vi "DAQ-Data-to-File Load Configuration Settings from XML.vi"(8 "error in (no error)":errorcluster, 11 "User Configuration in":T1={"Hardware Configuration"={"HW Refnum <Replace Me>"="", "Signal Type <Replace Me>"=enum."Sine Wave"}, "Analysis Configuration"={"Statistics"=TRUE}, "New Data Behavior"=enum."Replace"}) -> (0 "error out":errorcluster, 3 "User Configuration out":T1={"Hardware Configuration"={"HW Refnum <Replace Me>"="", "Signal Type <Replace Me>"=enum."Sine Wave"}, "Analysis Configuration"={"Statistics"=TRUE}, "New Data Behavior"=enum."Replace"})   [LabVIEW 2020]
doc: "Attempts to load previous user specified settings from an XML file.\n\nThis VI will not generate an error. If a suitable XML file can't be loaded and parsed then it will simply return the default settings."
uses:
  controls/DAQ-Data-to-File User Specified Data.ctl
  controls/DAQ-Data-to-File HW Configuration.ctl
  controls/DAQ-Data-to-File Simulated Signal Type.ctl
  controls/DAQ-Data-to-File Analysis Configuration.ctl
  controls/DAQ-Data-to-File New Data Behavior.ctl
  <vilib>/Utility/xml.llb/Read From XML File(string).vi
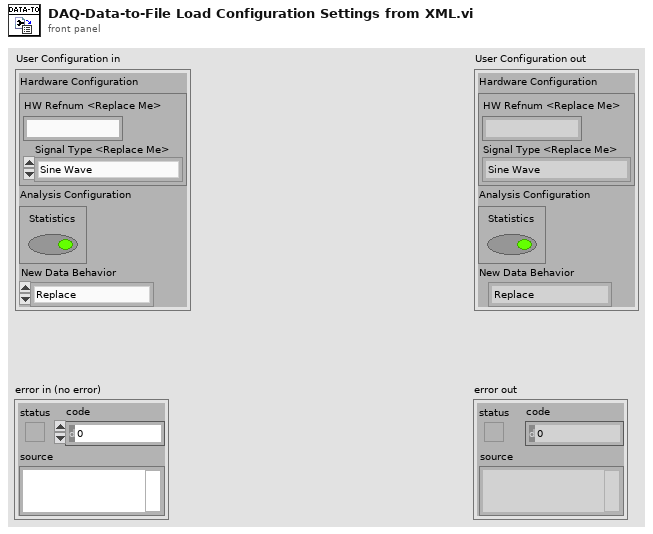
[diagram p1: front panel]
types:
  T1 = typedef "DAQ-Data-to-File User Specified Data.ctl" = cluster{"Hardware Configuration":T2, "Analysis Configuration":T4, "New Data Behavior":T5}
  T2 = typedef "DAQ-Data-to-File HW Configuration.ctl" = cluster{"HW Refnum <Replace Me>":string, "Signal Type <Replace Me>":T3}
  T3 = typedef "DAQ-Data-to-File Simulated Signal Type.ctl" = enum16{"Sine Wave", "Square Wave"}
  T4 = typedef "DAQ-Data-to-File Analysis Configuration.ctl" = cluster{"Statistics":bool}
  T5 = typedef "DAQ-Data-to-File New Data Behavior.ctl" = enum16{"Replace", "Overlay", "Append"}
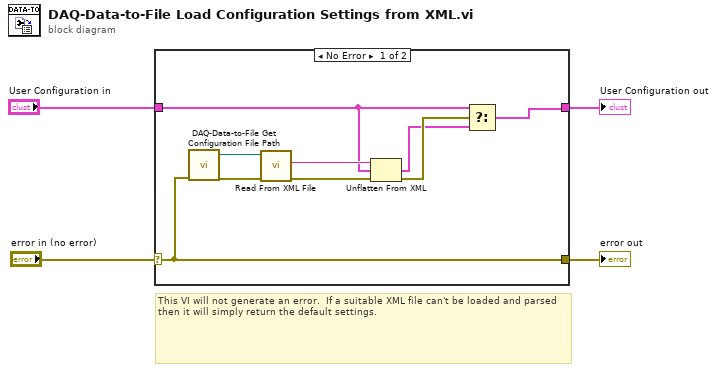
[diagram p0: block diagram]
diagram:
  # "This VI will not generate an error.  If a suitable XML file can't be loaded and parsed then it will simply return the default settings."
  n1 = case shown="No Error" "error in (no error)" {
    selector: "error in (no error)" -> [w10 w15]
    tunnel: [w10 w15] -> w3
    tunnel: "User Configuration in" -> [w7 w14]
    tunnel: [w5 w14] -> w1
    frame No Error {
      n2 = call "DAQ-Data-to-File Get Configuration File Path.vi"("error in (no error)"=w10) -> ("error out"=w12:errorcluster, "XML File Path"=w13:path)  [unwired: 9 in]
      n3 = call-poly <vilib>:"Read From XML File.vi"("error in (no error)"=w12, "XML File Path"=w13) -> ("error out"=w9:errorcluster, "XML Elements"=w11:string)  [unwired: 7 in, 1 out]
      n4 = Unflatten From XML(xml string=w11, type=w7, error in (no error)=w9) -> (value=w6:T1, error out=w8:errorcluster)
      n5 = Select(t=w7, s=w8, f=w6) -> (s? t:f=w5:T1)
    }
    frame Error {
    }
  }
  "error out" <- w3
  "User Configuration out" <- w1
